vi "Update MetaData Details.vi"(8 "error in":errorcluster, 11 "MeasurementService.lvclass":refnum<class "MeasurementService.lvclass">) -> (0 "error out":errorcluster, 3 "MeasurementService.lvclass":refnum<class "MeasurementService.lvclass">)   [LabVIEW 2020, in "LoadRegulation.lvlib"]
uses:
  LoadRegulation.lvlib
  RPC Service/MeasurementService/MeasurementService.lvclass
  C:/Program Files/National Instruments/LabVIEW 2020/vi.lib/gRPC/LabVIEW gRPC Servicer/ServiceBase/ServiceBase.lvclass
  RPC Messages/ni_measurements_v1_MeasurementParameters.ctl
  RPC Messages/ni_measurements_v1_ConfigurationParameter.ctl
  RPC Messages/google_protobuf_Any.ctl
  RPC Messages/ni_measurements_v1_Output.ctl
  Measurement Results.ctl
  Measurement Configuration.ctl
  RPC Service/MeasurementService/MeasurementService.lvclass/MeasurementService.ctl
  a3bfba1f-60ec-4a91-850f-cd9d7ba2e651.vi
  RPC Service/MeasurementService/Accessor/Write MeasurementDetails.vi
  RPC Service/MeasurementService/Accessor/Write MeasurementParameters.vi
  RPC Service/MeasurementService/Accessor/Write UserInterfaceDetails.vi
  <vilib>/gRPC/LabVIEW gRPC Library/Server API/Server/Get Server DLL Path.vi
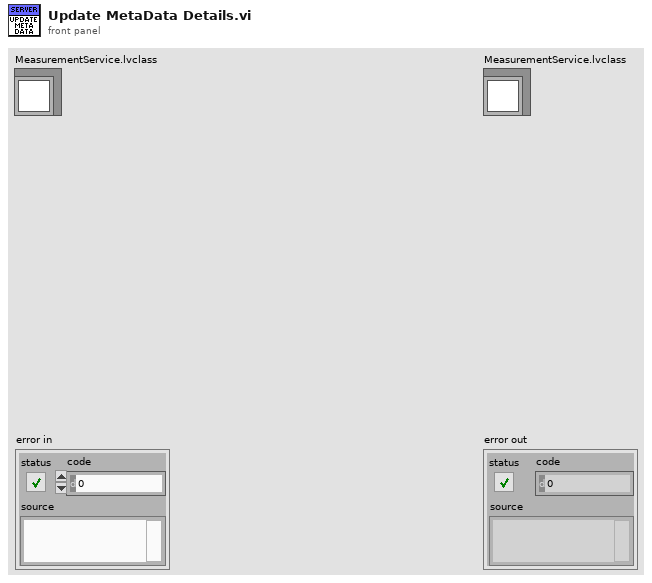
[diagram p1: front panel]
types:
  T1 = typedef "LoadRegulation.lvlib/ni_measurements_v1_MeasurementParameters.ctl" = cluster{"configuration_parameters_messagetype":string, "configuration_parameters":T2[], "configuration_defaults":T3, "outputs_message_type":string, "outputs":T4[]}
  T2 = typedef "LoadRegulation.lvlib/ni_measurements_v1_ConfigurationParameter.ctl" = cluster{"protobuf_id":u32, "type":i32, "name":string, "repeated":bool}
  T3 = typedef "LoadRegulation.lvlib/google_protobuf_Any.ctl" = cluster{"type_url":string, "value":u8[]}
  T4 = typedef "LoadRegulation.lvlib/ni_measurements_v1_Output.ctl" = cluster{"protobuf_id":u32, "type":i32, "name":string, "repeated":bool}
  T5 = typedef "LoadRegulation.lvlib/Measurement Configuration.ctl" = cluster{"Input Voltage in V":dbl, "Nominal Output Voltage in V":dbl, "Start":dbl, "Stop":dbl, "Step":dbl, "Input SMU":string, "Load SMU":string, "Input DMM":string, "Load DMM":string}
  T6 = typedef "LoadRegulation.lvlib/Measurement Results.ctl" = cluster{"Load Regulation (%)":dbl, "Load Regulation (mV/mA)":dbl, "Test Results.Load Current in A":dbl[], "Output Voltage in V":dbl[]}
  T7 = typedef "LoadRegulation.lvlib/ni_measurements_v1_MeasurementDetails.ctl" = cluster{"display_name":string, "version":string, "measurement_type":string, "product_type":string}
  T8 = typedef "gprc-lvsupport-release.lvlib/grpcId.ctl" = u64
  T9 = typedef "gprc-lvsupport-release.lvlib/Any.ctl" = cluster{"Type Url":string, "Bytes":u8[]}
  T10 = typedef "LoadRegulation.lvlib/ni_measurements_v1_UserInterfaceDetails.ctl" = cluster{"configuration_ui_url":string}
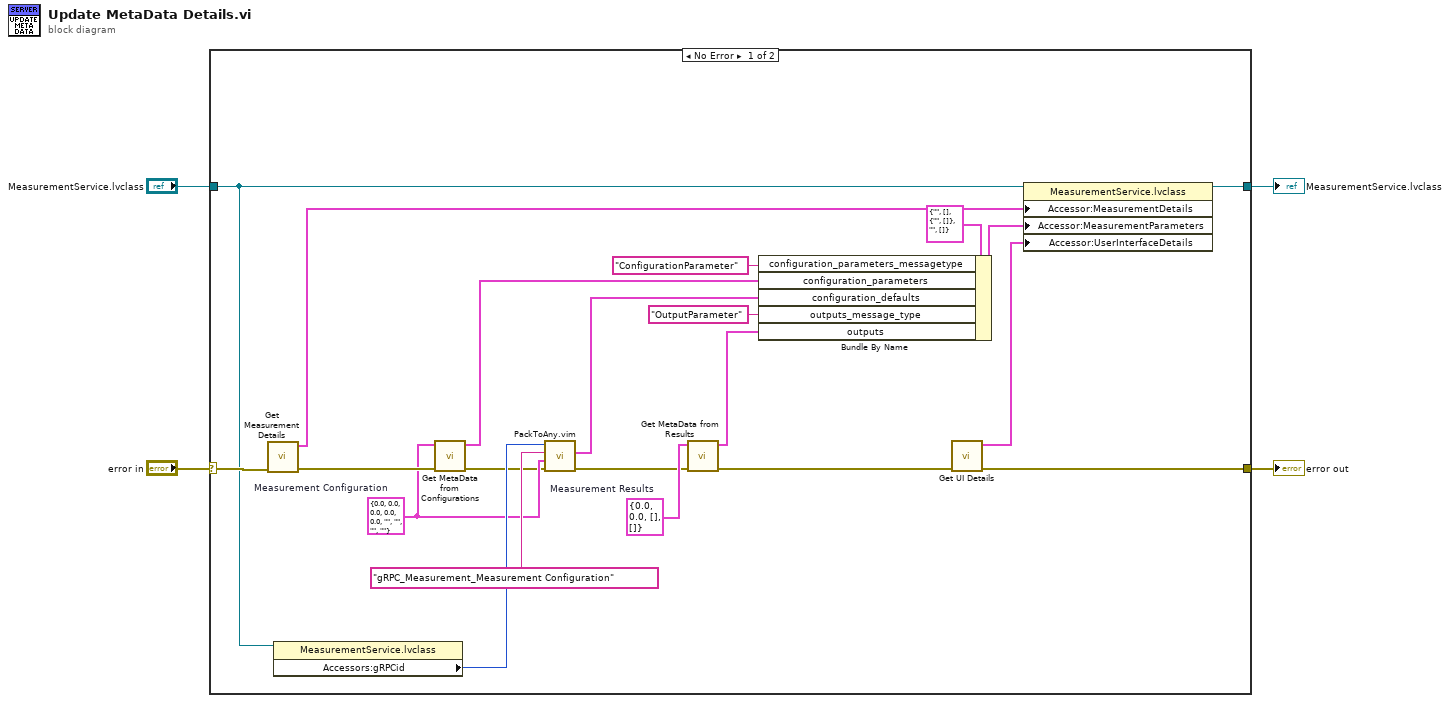
[diagram p0: block diagram]
diagram:
  n1 = case shown="No Error" "error in" {
    selector: "error in" -> [w25 w27]
    tunnel: [w5 w27] -> w3
    tunnel: "MeasurementService.lvclass" -> [w13 w26]
    tunnel: [w24 w26] -> w1
    frame No Error {
      w11 = T5 {"Input Voltage in V"=0.0, "Nominal Output Voltage in V"=0.0, "Start"=0.0, "Stop"=0.0, "Step"=0.0, "Input SMU"="", "Load SMU"="", "Input DMM"="", "Load DMM"=""}  # Measurement Configuration
      w17 = T6 {"Load Regulation (%)"=0.0, "Load Regulation (mV/mA)"=0.0, "Test Results.Load Current in A"=[], "Output Voltage in V"=[]}  # Measurement Results
      n2 = call "Get Measurement Details.vi"("error in"=w25) -> ("error out"=w20:errorcluster, "measurement_details"=w23:T7)  [unwired: 8 in, 1 out]
      n3 = property class="MeasurementService.lvclass"(reference=w13) -> ("Accessors:gRPCid"=w12:T8)  [unwired: 1 in, 2 out]
      n4 = call "Get MetaData from Configurations.vi"("error in"=w20, "Configuration Cluster"=w11) -> ("error out"=w10:errorcluster, "configuration_parameters"=w19:T2[])  [unwired: 8 in]
      n5 = call "PackToAny.vim"("error in (no error)"=w10, "Data To Pack"=w11, "Message Type"="gRPC_Measurement_Measurement Configuration", "gRPCid in"=w12) -> ("error out"=w9:errorcluster, "Any"=w8:T9)  [unwired: 5 in, 1 out]
      n6 = call "Get MetaData from Results.vi"("error in"=w9, "Configuration Cluster"=w17) -> ("error out"=w7:errorcluster, "outputs"=w18:T4[])  [unwired: 8 in]
      n7 = Bundle By Name(cluster=T1 {"configuration_parameters_messagetype"="", "configuration_parameters"=[], "configuration_defaults"={"type_url"="", "value"=[]}, "outputs_message_type"="", "outputs"=[]} ("MeasurementParameters"), "configuration_parameters_messagetype"="ConfigurationParameter", "configuration_parameters"=w19, "configuration_defaults"=w8, "outputs_message_type"="OutputParameter" ("configuration_parameters_messagetype"), "outputs"=w18) -> (w21:T1)
      n8 = call "Get UI Details.vi"("error in"=w7) -> ("error out"=w5:errorcluster, "UserInterfaceDetails"=w6:T10)  [unwired: 9 in]
      n9 = property class="MeasurementService.lvclass"(reference=w13, "Accessor:MeasurementDetails"=w23, "Accessor:MeasurementParameters"=w21, "Accessor:UserInterfaceDetails"=w6) -> (reference out=w24:refnum<class "MeasurementService.lvclass">)  [unwired: 1 in, 1 out]
    }
    frame Error {
    }
  }
  "MeasurementService.lvclass" <- w1
  "error out" <- w3
